vi "Search 1D Array Function.vi"() -> ()   [LabVIEW 2014]
panel:
  out "Index of element":i32
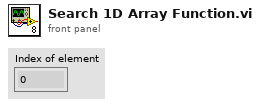
[diagram p1: front panel]
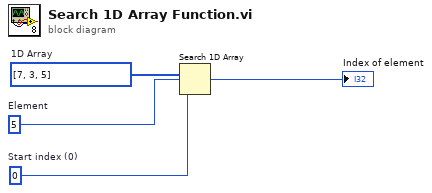
[diagram p0: block diagram]
diagram:
  w3 = 0  # Start index (0)
  w2 = 5  # Element
  w4 = i32[] [7, 3, 5]  # 1D Array
  n1 = Search 1D Array(1D array=w4, element=w2, start index (0)=w3) -> (index of element=→"Index of element":i32)
